vi "未命名 3.vi"() -> ()   [LabVIEW 2013]
uses:
  <vilib>/Utility/config.llb/NI_LVConfig.lvlib
panel:
  out "file created?":bool caption="文件已创建？"
  out "section names":string[](array[string]) caption="段名"
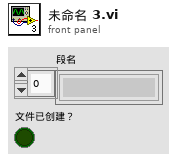
[diagram p1: front panel]
types:
  T1 = typedef "NI_LVConfig.lvlib/Config Data RefNum.ctl" = refnum<k1>
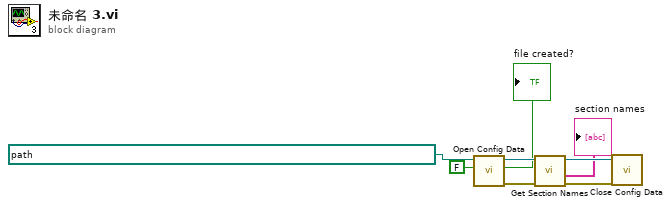
[diagram p0: block diagram]
diagram:
  n1 = call <vilib>:"Open Config Data.vi"("create file if necessary (T)"=FALSE, "configuration file path"=path "D:/BOOK/功能块/设计模式与项目模板/组件/跑马灯组件/data/跑马灯组件.ini") -> ("error out"=w6:errorcluster, "file created?"=→"file created?":bool, "refnum"=w5:T1)  [unwired: 7 in]
  n2 = call <vilib>:"Get Section Names.vi"("error in (no error)"=w6, "refnum"=w5) -> ("error out"=w3:errorcluster, "section names"=→"section names":string[], "refnum out"=w4:T1)  [unwired: 7 in]
  n3 = call <vilib>:"Close Config Data.vi"("error in (no error)"=w3, "refnum"=w4) -> ()  [unwired: 8 in, 2 out]
